vi "Schedule Flush.vi"(8 "error in":errorcluster, 11 "Report Generator in":refnum<class "Report Generator.lvclass">) -> (0 "error out":errorcluster, 3 "Report Generator out":refnum<class "Report Generator.lvclass">)   [LabVIEW 2023, in "Report Generator.lvlib" / "Report Generator.lvclass"]
uses:
  Library/Report Generator.lvclass
  C:/Users/Public/Documents/Development/builds/Engine/Engine.lvlibp/Project/Engine.lvclass
  Report Generator Messages/Periodic Flush Queue Msg/Periodic Flush Queue Msg.lvclass
  C:/Users/Public/Documents/Development/builds/Engine/Actor Framework.lvlibp/1abvi3w/vi.lib/ActorFramework/Message/Message.lvclass
  Library/Report Generator.lvclass/Report Generator.ctl
  builds/Engine/Engine.lvlibp/Accessors/Read Self Q.vi
  builds/Engine/Actor Framework.lvlibp/1abvi3w/vi.lib/ActorFramework/Message Enqueuer/Message Enqueuer.lvclass
  builds/Engine/Actor Framework.lvlibp
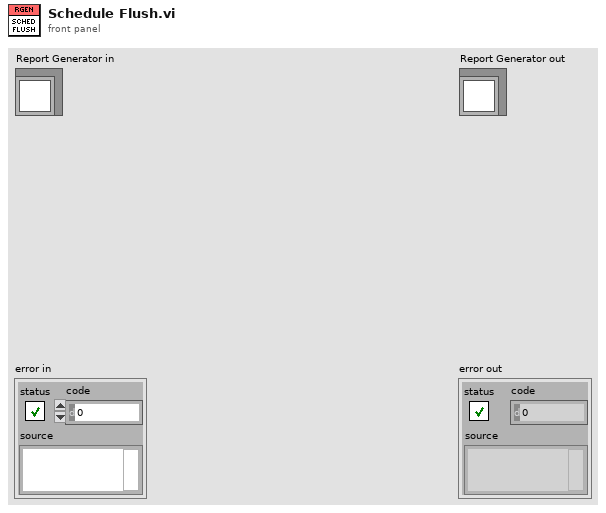
[diagram p1: front panel]
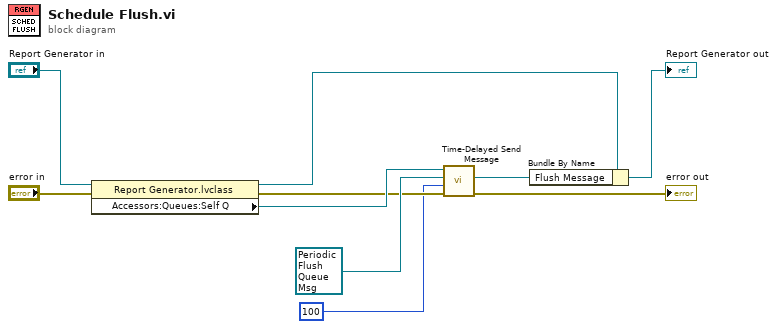
[diagram p0: block diagram]
diagram:
  n1 = property class="Report Generator.lvclass"(reference="Report Generator in", error in="error in") -> (reference out=w2:refnum<class "Report Generator.lvclass">, error out=w4:errorcluster, "Accessors:Queues:Self Q"=w6:refnum<class "Message Enqueuer.lvclass">)
  n2 = call "Time-Delayed Send Message.vi"("error in (no error)"=w4, "Milliseconds To Wait"=100, "Message"=refnum<class "Periodic Flush Queue Msg.lvclass"> refnum ("Report Generator.lvlib:Periodic Flush Queue Msg.lvclass"), "Message Enqueuer"=w6) -> ("error out"=→"error out":errorcluster, "Delivery Notifier"=w10:refnum<notifier>)  [unwired: 6 in]
  n3 = Bundle By Name(cluster=w2, "Flush Message"=w10) -> (→"Report Generator out":refnum<class "Report Generator.lvclass">)
